vi "Gen2 FT Globals.vi"() -> ()   [LabVIEW 2015]
panel:
  out "Transceiver Ch":refnum<vi>
  out "Page Num":refnum<vi>
  in  "Device Reset?":bool
  in  "CustomCalFactors?":bool
  in  "DeviceType":u16
  in  "RawRxTx":bool
  in  "ZeroDev?":bool
  in  "BaseCalA/D":u16
  in  "BattCal A/Ds":dbl[](array[numeric])
  in  "BattCal Volts":dbl[](array[numeric])
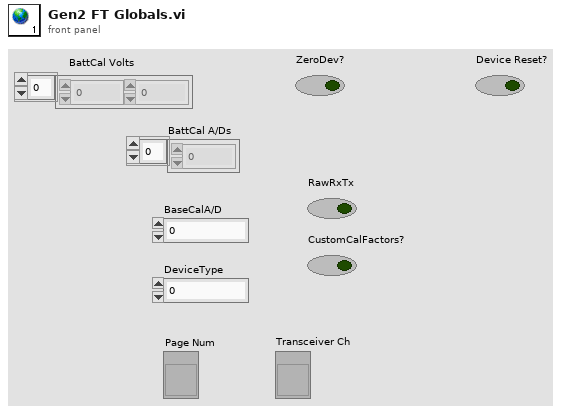
[diagram p1: front panel]
diagram:
